vi "solar_cfg Simple (Sections).vi"(8 "error in (no error)":errorcluster, 9 "Keys":string[](array[string]), 10 "Section":string, 11 "Config Path (*.ini)":path) -> (0 "error out":errorcluster, 1 "Values":string[](array[string]), 2 "Sections":cluster{"Section":string, "kvc":string[][]}[](array[cluster]), 3 "dup Config Path":path)   [LabVIEW 2018]
doc: "This VI reads or writes a single item from a configuration file. The key is created if not found."
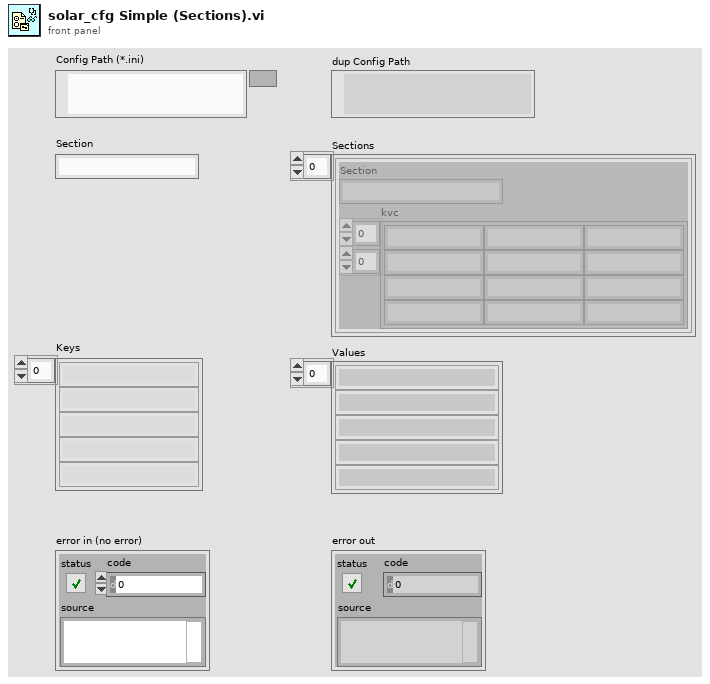
[diagram p1: front panel]
types:
  T1 = enum16{"open", "replace", "create", "open or create", "replace or create", "replace or create with confirmation"}
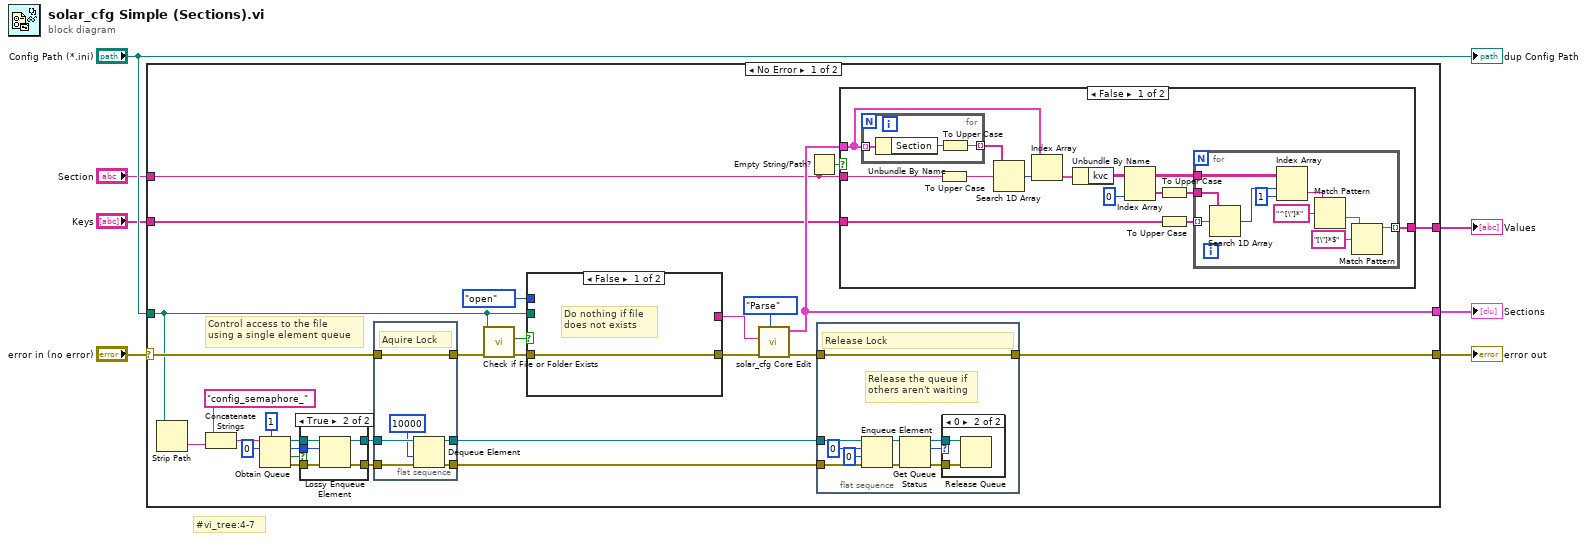
[diagram p0: block diagram]
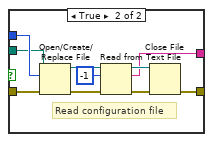
[diagram p2: hidden frame]
diagram:
  # "#vi_tree:4-7"
  n1 = case shown="No Error" "error in (no error)" {
    selector: "error in (no error)" -> [w23 w98]
    tunnel: "Config Path (*.ini)" -> [w9 _]
    tunnel: [w17 w98] -> w6
    tunnel: [w15 _] -> w4
    tunnel: "Keys" -> [w14 _]
    tunnel: "Section" -> [w12 _]
    tunnel: [w13 _] -> w1
    frame No Error {
      w26 = u8 0
      # "Control access to the file\nusing a single element queue"
      n2 = Strip Path(path=w9) -> (name=w21:string)  [unwired: 1 out]
      n3 = Concatenate Strings("config_semaphore_" ("string"), w21) -> (w28:string)
      n4 = Obtain Queue(max queue size (-1, unlimited)=1, name (unnamed)=w28, element data type=w26) -> (queue out=w31:refnum<queue>, created new?=w32:bool, error out=w30:errorcluster)  [unwired: 2 in]
      n5 = case shown="True" w32 {
        tunnel: w31 -> [w92 w97]
        tunnel: w30 -> [w91 w96]
        tunnel: w26 -> [_ w95]
        tunnel: [w92 w94] -> w29
        tunnel: [w91 w93] -> w25
        frame False {
        }
        frame True {
          n6 = Lossy Enqueue Element(queue=w97, element=w95, error in (no error)=w96) -> (queue out=w94:refnum<queue>, error out=w93:errorcluster)  [unwired: 2 out]
        }
      }
      n7 = flat-sequence {
        tunnel: [w90] -> w34
        tunnel: w29 -> [w89]
        tunnel: w25 -> [w88]
        tunnel: [w86] -> w24
        tunnel: w23 -> [w86]
        tunnel: [w85] -> w22
        frame #0 {
          # "Aquire Lock"
          n8 = Dequeue Element(queue=w89, timeout in ms (-1)=10000, error in (no error)=w88) -> (queue out=w90:refnum<queue>, error out=w85:errorcluster)  [unwired: 2 out]
        }
      }
      n9 = call <vilib>:"Check if File or Folder Exists.vi"("error in (no error)"=w24, "path"=w9) -> ("error out"=w10:errorcluster, "file or folder exists?"=w8:bool)  [unwired: 7 in, 1 out]
      n10 = case shown="False" w8 {
        tunnel: T1."open" ("operation (0:open)") -> [_ w41]
        tunnel: w10 -> [w36 w40]
        tunnel: [w36 w39] -> w20
        tunnel: [_ w38] -> w19
        tunnel: w9 -> [_ w37]
        frame False {
          # "Do nothing if file \ndoes not exists"
        }
        frame True {
          # "Read configuration file"
          n11 = Open/Create/Replace File(file path (use dialog)=w37, error in=w40, operation (0:open)=w41) -> (refnum out=w42:refnum<file>, error out=w43:errorcluster)  [unwired: 3 in, 1 out]
          n12 = Read from Text File(file (use dialog)=w42, count=-1, error in=w43) -> (refnum out=w45:refnum<file>, text=w38:string, error out=w46:errorcluster)  [unwired: 1 in, 1 out]
          n13 = Close File(refnum=w45, error in=w46) -> (error out=w39:errorcluster)  [unwired: 1 out]
        }
      }
      n14 = call "solar_cfg Core Edit.vi"("Action (Read)"=enum8{"Read", "Write", "Parse", "Build"}."Parse", "error in (no error)"=w20, "Section/String in"=w19) -> ("error out"=w16:errorcluster, "Sections out"=w15:cluster{"Section":string, "kvc":string[][]}[])  [unwired: 4 in, 3 out]
      n15 = Empty String/Path?(string/path=w12) -> (empty?=w11:bool)
      n16 = flat-sequence {
        tunnel: w34 -> [w82]
        tunnel: w22 -> [w79]
        tunnel: [w73] -> w17
        tunnel: w16 -> [w73]
        frame #0 {
          # "Release the queue if\nothers aren't waiting"
          # "Release Lock"
          n17 = Enqueue Element(queue=w82, element=u8 0, timeout in ms (-1)=0, error in (no error)=w79) -> (queue out=w75:refnum<queue>, error out=w74:errorcluster)  [unwired: 1 out]
          n18 = Get Queue Status(queue=w75, error in (no error)=w74) -> (queue out=w77:refnum<queue>, # pending remove=w76:i32, error out=w78:errorcluster)  [unwired: 1 in, 5 out]
          n19 = case shown="0" w76 {
            tunnel: w77 -> [_ w84]
            tunnel: w78 -> [_ w83]
            frame Default {
            }
            frame 0 {
              n20 = Release Queue(queue=w84, error in (no error)=w83) -> ()  [unwired: 1 in, 3 out]
            }
          }
        }
      }
      n21 = case shown="False" w11 {
        tunnel: w15 -> [w50 _]
        tunnel: w14 -> [w49 _]
        tunnel: w12 -> [w48 _]
        tunnel: [w47 _] -> w13
        frame False {
          n22 = for {
            tunnel: w50 -> [w72] mode=indexing
            tunnel: [w70] -> w59 mode=indexing
            n23 = Unbundle By Name(w72) -> ("Section"=w71:string)
            n24 = To Upper Case(1:w71) -> (0:w70:string)
          }
          n25 = To Upper Case(1:w48) -> (0:w51:string)
          n26 = Search 1D Array(1D array=w59, element=w51) -> (index of element=w58:i32)  [unwired: 1 in]
          n27 = Index Array(array=w50, index=w58) -> (element=w57:cluster{"Section":string, "kvc":string[][]})
          n28 = Unbundle By Name(w57) -> ("kvc"=w53:string[][])
          n29 = Index Array(array=w53, index (col)=0 ("disabled index (col)")) -> (element=w55:string[])  [unwired: 1 in]
          n30 = To Upper Case(1:w55) -> (0:w54:string[])
          n31 = To Upper Case(1:w49) -> (0:w52:string[])
          n32 = for {
            tunnel: w54 -> [w69]
            tunnel: w52 -> [w68] mode=indexing
            tunnel: w53 -> [w67]
            tunnel: [w60] -> w47 mode=indexing
            n33 = Search 1D Array(1D array=w69, element=w68) -> (index of element=w66:i32)  [unwired: 1 in]
            n34 = Index Array(array=w67, index (row)=w66, index (col)=1 ("disabled index (col)")) -> (element=w61:string)
            n35 = Match Pattern(string=w61, regular expression="^[\"]*") -> (after substring=w62:string)  [unwired: 1 in, 3 out]
            n36 = Match Pattern(string=w62, regular expression="[\"]*$") -> (before substring=w60:string)  [unwired: 1 in, 3 out]
          }
        }
        frame True {
        }
      }
    }
    frame Error {
    }
  }
  "error out" <- w6
  "Sections" <- w4
  "Values" <- w1
  "dup Config Path" <- "Config Path (*.ini)"
